vi "ExposeMapperToObjectNamepathData.vi"(8 "BaseName":string, 9 "Skip Parent Name (t)":bool=TRUE, 10 "Value Reference In":refnum<data-value>, 11 "Value":variant) -> (3 "Object map":T1[](array[typedef]))   [LabVIEW 2017]
uses:
  ExposeObjectMapNamepathData.ctl
  ExposeMapperDataTypeEnum.ctl
  ExposeObjectMapContainerTypeEnum.ctl
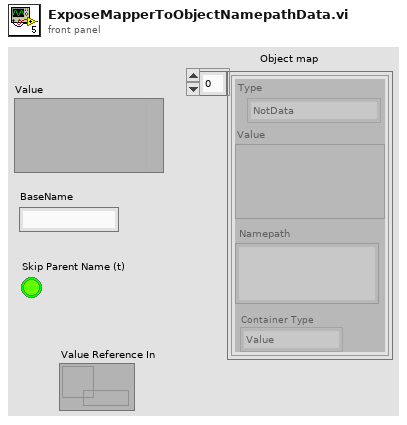
[diagram p1: front panel]
types:
  T1 = typedef "ExposeObjectMapNamepathData.ctl" = cluster{"Type":T2, "Value":variant, "Namepath":string, "Container Type":T3}
  T2 = typedef "ExposeMapperDataTypeEnum.ctl" = enum16{"NotData", "int8", "byte", "int16", "uint16", "int32", "uint32", "int64", "uint64", "Single", "Double", "String", "Boolean", "Container"}
  T3 = typedef "ExposeObjectMapContainerTypeEnum.ctl" = enum16{"Value", "Array", "Waveform", "NetContainer"}
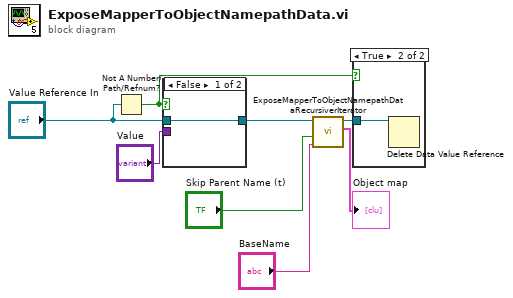
[diagram p0: block diagram]
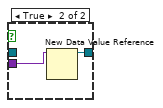
[diagram p3: hidden frame]
diagram:
  n1 = Not A Number/Path/Refnum?(number/path/refnum="Value Reference In") -> (NaN/Path/Refnum?=w2:bool)
  n2 = case shown="False" w2 {
    tunnel: "Value" -> [_ w11]
    tunnel: [w9 w10] -> w4
    tunnel: "Value Reference In" -> [w9 _]
    frame False {
    }
    frame True {
      n3 = New Data Value Reference(data value=w11) -> (data value reference=w10:refnum<data-value>)  [unwired: 1 in, 1 out]
    }
  }
  n4 = call "ExposeMapperToObjectNamepathDataRecursiverIterator.vi"("BaseName"="BaseName", "Skip Parent Name (t)"="Skip Parent Name (t)", "Value Reference In"=w4) -> ("Object map"=→"Object map":T1[], "Value Reference Out"=w1:refnum<data-value>)  [unwired: 7 in]
  n5 = case shown="True" w2 {
    tunnel: w1 -> [_ w12]
    frame False {
    }
    frame True {
      n6 = Delete Data Value Reference(data value reference=w12) -> ()  [unwired: 1 in, 2 out]
    }
  }
